vi "smallCarTemp.vi"(6 "time_frame":cluster{"secs":i32, "nsecs":i32}, 8 "error_message":string, 9 "error":i8, 10 "set_steering":dbl, 11 "set_speed":dbl) -> (3 "msg out":string)   [LabVIEW 2016]
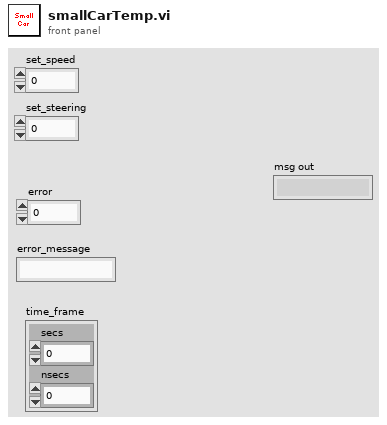
[diagram p1: front panel]
types:
  T1 = cluster{"front_left":dbl, "front_right":dbl, "back_left":dbl, "back_right":dbl}
  T2 = cluster{"speed_is":cluster{"front_left":dbl, "front_right":dbl, "back_left":dbl, "back_right":dbl}, "steering_is":cluster{"front_left":dbl, "front_right":dbl, "back_left":dbl, "back_right":dbl}, "error":i8, "error_message":string, "time":cluster{"secs":i32, "nsecs":i32}}
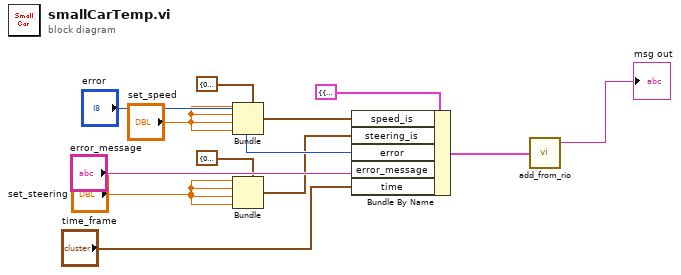
[diagram p0: block diagram]
diagram:
  n1 = Bundle(cluster=T1 {"front_left"=0.0, "front_right"=0.0, "back_left"=0.0, "back_right"=0.0} ("speed_is"), "front_left"="set_speed", "front_right"="set_speed", "back_left"="set_speed", "back_right"="set_speed") -> (w10:T1)
  n2 = Bundle(cluster=T1 {"front_left"=0.0, "front_right"=0.0, "back_left"=0.0, "back_right"=0.0} ("speed_is"), "front_left"="set_steering", "front_right"="set_steering", "back_left"="set_steering", "back_right"="set_steering") -> (w7:T1)
  n3 = Bundle By Name(cluster=T2 {"speed_is"={"front_left"=0.0, "front_right"=0.0, "back_left"=0.0, "back_right"=0.0}, "steering_is"={"front_left"=0.0, "front_right"=0.0, "back_left"=0.0, "back_right"=0.0}, "error"=0, "error_message"="", "time"={"secs"=0, "nsecs"=0}} ("from_rio"), "speed_is"=w10, "steering_is"=w7, "error"="error", "error_message"="error_message", "time"="time_frame") -> (w3:T2)
  n4 = call "add_from_rio.vi"("from_rio"=w3) -> ("msg out"=→"msg out":string)  [unwired: 4 in]
